vi "String To Dbl.vi"(11 "String":string) -> (3 "Numeric":dbl)   [LabVIEW 2019]
panel:
  # "converte stringa in numero\ntenendo conto del separatore \ndecimale di sistema"
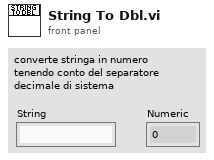
[diagram p1: front panel]
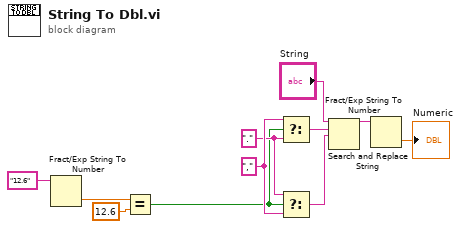
[diagram p0: block diagram]
diagram:
  w6 = "."
  w8 = ","
  n1 = Fract/Exp String To Number(string="12.6") -> (number=w1:dbl)  [unwired: 3 in, 1 out]
  n2 = Equal?(x=w1, y=12.6) -> (x = y?=w4:bool)
  n3 = Select(t=w8, s=w4, f=w6) -> (s? t:f=w5:string)
  n4 = Select(t=w6, s=w4, f=w8) -> (s? t:f=w7:string)
  n5 = Search and Replace String(input string="String", search string=w5, replace string=w7) -> (result string=w9:string)  [unwired: 5 in, 3 out]
  n6 = Fract/Exp String To Number(string=w9) -> (number=→"Numeric":dbl)  [unwired: 3 in, 1 out]
